vi "SoC.vi"(0 "BAT Current (A)":dbl, 1 "Coefficients":dbl[](array[numeric])) -> (2 "SoC (%)":i32, 3 "State":string, 4 "Time (min)":i32)   [LabVIEW 2015]
uses:
  <vilib>/Analysis/polynomials.llb/Polynomial Roots (DBL).vi
  <vilib>/Analysis/NI_AALPro.lvlib
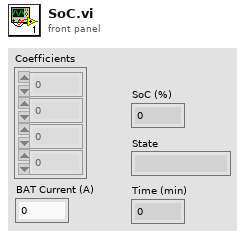
[diagram p1: front panel]
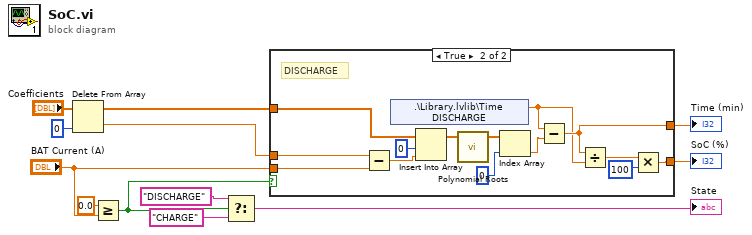
[diagram p0: block diagram]
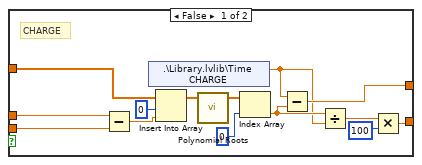
[diagram p2: hidden frame]
diagram:
  n1 = Delete From Array(array="Coefficients", index=0) -> (deleted portion=w2:dbl, array with subset deleted=w3:dbl[])  [unwired: 1 in]
  n2 = Greater Or Equal?(x=0.0, y="BAT Current (A)") -> (x >= y?=w9:bool)
  n3 = Select(t="DISCHARGE" ("f"), s=w9, f="CHARGE" ("t")) -> (s? t:f=→"State":string)
  n4 = case shown="True" w9 {
    tunnel: [w19 w32] -> w6
    tunnel: [w18 w31] -> w7
    tunnel: "BAT Current (A)" -> [w16 w30]
    tunnel: w3 -> [w15 w29]
    tunnel: w2 -> [w14 w28]
    frame False {
      # "CHARGE"
      n5 = Subtract(x=w14, y=w16) -> (x-y=w21:dbl)
      n6 = shared-variable ".\\Library.lvlib\\Time CHARGE"() -> (w13:dbl)  [unwired: 1 in, 1 out]
      n7 = Insert Into Array(array=w15, index=0, new element=w21) -> (w20:dbl[])
      n8 = call-poly <vilib>:"Polynomial Roots.vi"("P(x)"=w20) -> ("Roots"=w26:cdb[])  [unwired: 9 in, 1 out]
      n9 = Index Array(array=w26, index=0) -> (element=w17:cdb)
      n10 = Subtract(x=w13, y=w17) -> (x-y=w19:cdb)
      n11 = Divide(x=w17, y=w13) -> (x/y=w25:cdb)
      n12 = Multiply(x=w25, y=100) -> (x*y=w18:cdb)
    }
    frame True {
      # "DISCHARGE"
      n13 = Subtract(x=w28, y=w30) -> (x-y=w34:dbl)
      n14 = shared-variable ".\\Library.lvlib\\Time DISCHARGE"() -> (w27:dbl)  [unwired: 1 in, 1 out]
      n15 = Insert Into Array(array=w29, index=0, new element=w34) -> (w33:dbl[])
      n16 = call-poly <vilib>:"Polynomial Roots.vi"("P(x)"=w33) -> ("Roots"=w36:cdb[])  [unwired: 9 in, 1 out]
      n17 = Index Array(array=w36, index=0) -> (element=w40:cdb)
      n18 = Subtract(x=w27, y=w40) -> (x-y=w32:cdb)
      n19 = Divide(x=w32, y=w27) -> (x/y=w39:cdb)
      n20 = Multiply(x=w39, y=100) -> (x*y=w31:cdb)
    }
  }
  "SoC (%)" <- w7
  "Time (min)" <- w6
